vi "Initialize DAQ Data.vi"(8 "error in (no error)":errorcluster, 11 "DAQ":refnum<class "DAQ.lvclass">) -> (0 "error out":errorcluster, 3 "DAQ":refnum<class "DAQ.lvclass">)   [LabVIEW 2017, in "DAQ.lvclass"]
doc: "Developed by Kevin Thompson\nkevin@thompsonengineering.net\n\nCopyright 2018-2020\nThompson Engineering, LLC"
uses:
  DAQ.lvclass
  DAQ.lvclass/DAQ.ctl
  DataTypes/TD AI TaskIO.ctl
  DataTypes/TD DI TaskIO.ctl
  Accessors/Get DO IONames.vi
  Accessors/Get DI TaskNames.vi
  Accessors/Get AO IONames.vi
  Accessors/Get DAQData Dict.vi
  Accessors/Get DAQNodes Dict.vi
  Accessors/Get AI TaskNames.vi
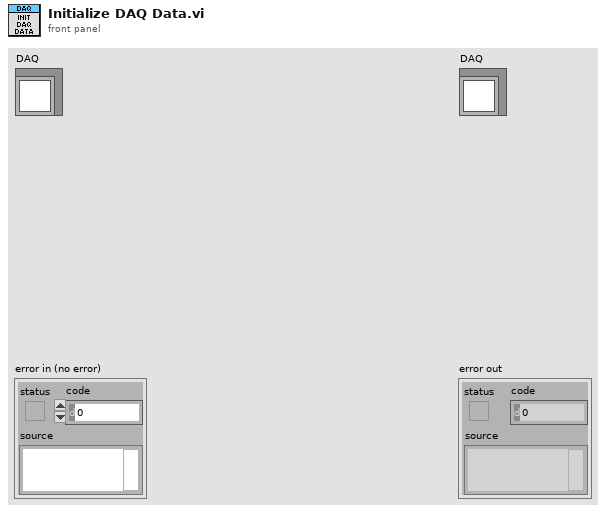
[diagram p1: front panel]
types:
  T1 = typedef "TD Dynamic CVT DVR--ref.ctl" = refnum<data-value>
  T2 = typedef "DAQ.lvclass/TD AI TaskIO.ctl" = cluster{"AI TaskName":string, "IONames":string[], "DAQmx AI TaskRef":refnum<k21>}
  T3 = typedef "DAQ.lvclass/TD DI TaskIO.ctl" = cluster{"DI TaskName":string, "IONames":string[], "DAQmxDI TaskRef":refnum<k21>}
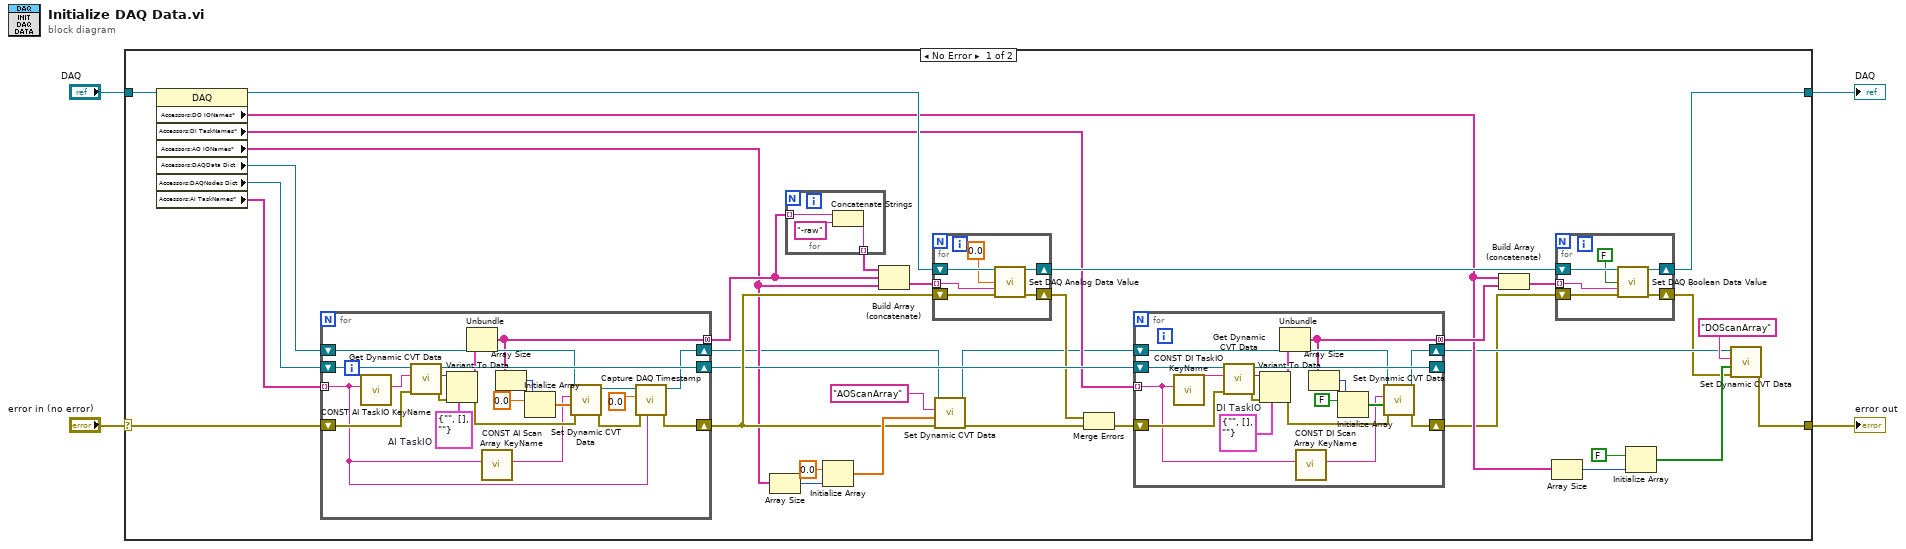
[diagram p0: block diagram]
diagram:
  n1 = case shown="No Error" "error in (no error)" {
    selector: "error in (no error)" -> [w24 w95]
    tunnel: [w6 w95] -> w3
    tunnel: [w38 w94] -> w1
    tunnel: "DAQ" -> [w29 w94]
    frame No Error {
      n2 = property class="DAQ"(reference=w29) -> (reference out=w25:refnum<class "DAQ.lvclass">, "Accessors:DO IONames*"=w17:string[], "Accessors:DI TaskNames*"=w16:string[], "Accessors:AO IONames*"=w18:string[], "Accessors:DAQData Dict"=w11:T1, "Accessors:DAQNodes Dict"=w10:T1, "Accessors:AI TaskNames*"=w9:string[])  [unwired: 1 in, 1 out]
      n3 = for {
        tunnel: w9 -> [w72] mode=indexing
        shift-right: [w68] -> w23
        shift-left: w24 -> [w80]
        shift-right: [w70] -> w7
        shift-left: w11 -> [w77]
        shift-right: [w78] -> w22
        shift-left: w10 -> [w87]
        tunnel: [w73] -> w26 mode=concatenating
        w74 = T2 {"AI TaskName"="", "IONames"=[], "DAQmx AI TaskRef"=""}  # AI TaskIO
        n4 = call "CONST AI TaskIO KeyName.vi"("AI TaskName"=w72) -> ("AI TaskIO (KeyName)"=w86:string)  [unwired: 10 in]
        n5 = call <vilib>:"Get Dynamic CVT Data.vi"("error in (no error)"=w80, "DataName"=w86, "dCVT DVR"=w87) -> ("error out"=w85:errorcluster, "value"=w84:variant, "dCVT DVR out"=w78:T1)  [unwired: 5 in, 1 out]
        n6 = Variant To Data(error in=w85, type=w74, Variant=w84) -> (data=w75:T2, error out=w79:errorcluster)
        n7 = Unbundle(w75) -> ("IONames"=w73:string[])  [unwired: 2 out]
        n8 = call "CONST AI Scan Array KeyName.vi"("AI TaskName"=w72) -> ("AI ScanArray (KeyName)"=w76:string)  [unwired: 10 in]
        n9 = Array Size(array=w73) -> (size(s)=w83:i32)
        n10 = Initialize Array(0.0, w83) -> (w81:dbl[])
        n11 = call <vilib>:"Set Dynamic CVT Data.vi"("error in (no error)"=w79, "value"=w81, "DataName"=w76, "dCVT DVR"=w77) -> ("error out"=w69:errorcluster, "dCVT DVR out"=w71:T1)  [unwired: 5 in, 1 out]
        n12 = call "Capture DAQ Timestamp.vi"("DaqData dCVT"=w71, "timestamp in"=0.0, "error in (no error)"=w69, "AI TaskName"=w72) -> ("DaqData dCVT out"=w70:T1, "error out"=w68:errorcluster)  [unwired: 4 in, 1 out]
      }
      n13 = Array Size(array=w18) -> (size(s)=w36:i32)
      n14 = for {
        tunnel: w26 -> [w60] mode=indexing
        tunnel: [w58] -> w27 mode=indexing
        n15 = Concatenate Strings(w60, "-raw" ("string")) -> (w58:string)
      }
      n16 = Initialize Array(0.0, w36) -> (w35:dbl[])
      n17 = Build Array (concatenate)(w27, w26, w18) -> (w28:string[])
      n18 = for {
        shift-right: [w63] -> w19
        shift-left: w25 -> [w66]
        shift-right: [w65] -> w14
        shift-left: w23 -> [w64]
        tunnel: w28 -> [w62] mode=indexing
        n19 = call "Set DAQ Analog Data Value.vi"("DAQ"=w66, "Value"=0.0, "Name"=w62, "error in (no error)"=w64) -> ("DAQ"=w63:refnum<class "DAQ.lvclass">, "error out"=w65:errorcluster)  [unwired: 9 in, 1 out]
      }
      n20 = call <vilib>:"Set Dynamic CVT Data.vi"("error in (no error)"=w23, "value"=w35, "DataName"="AOScanArray", "dCVT DVR"=w7) -> ("error out"=w21:errorcluster, "dCVT DVR out"=w8:T1)  [unwired: 5 in, 1 out]
      n21 = Merge Errors(w14, w21) -> (w13:errorcluster)
      n22 = for {
        tunnel: w16 -> [w41] mode=indexing
        shift-right: [w51] -> w12
        shift-left: w13 -> [w52]
        shift-right: [w47] -> w15
        shift-left: w8 -> [w48]
        shift-right: [w49] -> _
        shift-left: w22 -> [w57]
        tunnel: [w45] -> w20 mode=concatenating
        w43 = T3 {"DI TaskName"="", "IONames"=[], "DAQmxDI TaskRef"=""}  # DI TaskIO
        n23 = call "CONST DI TaskIO KeyName.vi"("DI TaskName"=w41) -> ("DI TaskIO (KeyName)"=w44:string)  [unwired: 10 in]
        n24 = call <vilib>:"Get Dynamic CVT Data.vi"("error in (no error)"=w52, "DataName"=w44, "dCVT DVR"=w57) -> ("error out"=w56:errorcluster, "value"=w55:variant, "dCVT DVR out"=w49:T1)  [unwired: 5 in, 1 out]
        n25 = Variant To Data(error in=w56, type=w43, Variant=w55) -> (data=w46:T3, error out=w50:errorcluster)
        n26 = Unbundle(w46) -> ("IONames"=w45:string[])  [unwired: 2 out]
        n27 = call "CONST DI Scan Array KeyName.vi"("DI TaskName"=w41) -> ("DI ScanArray (KeyName)"=w40:string)  [unwired: 10 in]
        n28 = Array Size(array=w45) -> (size(s)=w54:i32)
        n29 = Initialize Array(FALSE, w54) -> (w53:bool[])
        n30 = call <vilib>:"Set Dynamic CVT Data.vi"("error in (no error)"=w50, "value"=w53, "DataName"=w40, "dCVT DVR"=w48) -> ("error out"=w51:errorcluster, "dCVT DVR out"=w47:T1)  [unwired: 5 in, 1 out]
      }
      n31 = Build Array (concatenate)(w17, w20) -> (w39:string[])
      n32 = Array Size(array=w17) -> (size(s)=w32:i32)
      n33 = for {
        shift-right: [w90] -> w38
        shift-left: w19 -> [w93]
        shift-right: [w92] -> w5
        shift-left: w12 -> [w91]
        tunnel: w39 -> [w89] mode=indexing
        n34 = call "Set DAQ Boolean Data Value.vi"("DAQ"=w93, "Value"=FALSE, "Name"=w89, "error in (no error)"=w91) -> ("DAQ"=w90:refnum<class "DAQ.lvclass">, "error out"=w92:errorcluster)  [unwired: 9 in, 1 out]
      }
      n35 = Initialize Array(FALSE, w32) -> (w30:bool[])
      n36 = call <vilib>:"Set Dynamic CVT Data.vi"("error in (no error)"=w5, "value"=w30, "DataName"="DOScanArray", "dCVT DVR"=w15) -> ("error out"=w6:errorcluster)  [unwired: 5 in, 2 out]
    }
    frame Error {
    }
  }
  "error out" <- w3
  "DAQ" <- w1
